vi "数据标识判定.vi"(8 "通讯故障":bool, 9 "量程下限":dbl, 10 "量程上限":dbl, 11 "测量值":sgl) -> (3 "数据标识":string)   [LabVIEW 2016, in "斯坦道多参数.lvlib"]
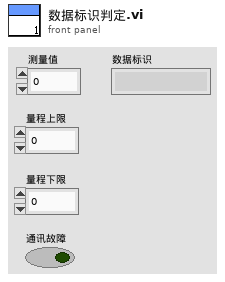
[diagram p1: front panel]
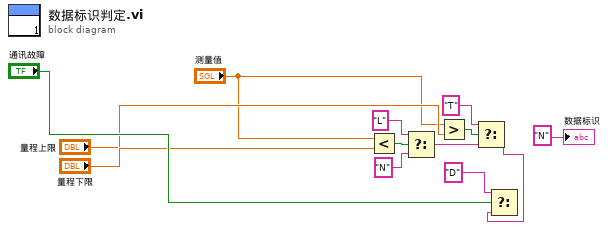
[diagram p0: block diagram]
diagram:
  n1 = Less?(x="测量值", y="量程下限") -> (x < y?=w7:bool)
  n2 = Select(t="L", s=w7, f="N") -> (s? t:f=w10:string)
  n3 = Greater?(x="测量值", y="量程上限") -> (0:w5:bool)
  n4 = Select(t="T", s=w5, f=w10) -> (s? t:f=w13:string)
  n5 = Select(t="D", s="通讯故障", f=w13) -> ()  [unwired: 1 out]
  "数据标识" <- "N"
